vi "Convert Units - Ratios.vi"(7 "units":T1, 10 "linear ratio":dbl) -> (2 "converted ratio":dbl)   [LabVIEW 2022 SP3]
uses:
  controls/measurement units.ctl
  <vilib>/addons/Sound and Vibration/svt_Distortion/SoundVib_Distortion.lvlib
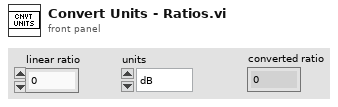
[diagram p1: front panel]
types:
  T1 = typedef "measurement units.ctl" = enum32{"dB", "%", "x/y"}
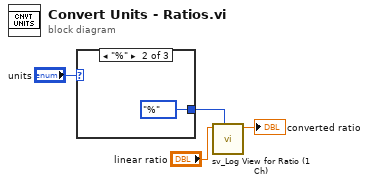
[diagram p0: block diagram]
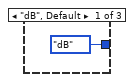
[diagram p2: hidden frame]
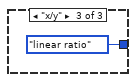
[diagram p3: hidden frame]
diagram:
  n1 = case shown="\"%\"" "units" {
    tunnel: [enum16{"dB", "linear ratio", "%"}."dB" ("ratio units") enum16{"dB", "linear ratio", "%"}."%" ("ratio units") enum16{"dB", "linear ratio", "%"}."linear ratio" ("ratio units")] -> w3
    frame "dB", Default {
    }
    frame "%" {
    }
    frame "x/y" {
    }
  }
  n2 = call <vilib>:"sv_Log View for Ratio (1 Ch).vi"("ratio units"=w3, "linear ratio"="linear ratio") -> ("converted ratio"=→"converted ratio":dbl)  [unwired: 7 in, 2 out]
